vi "GF_CheckIgnoreError.vi"(1 "error in":errorcluster, 2 "Error code to ignore":i32) -> (0 "error out":errorcluster)   [LabVIEW 2016]
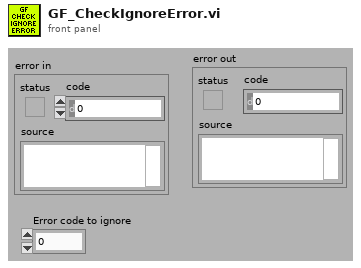
[diagram p1: front panel]
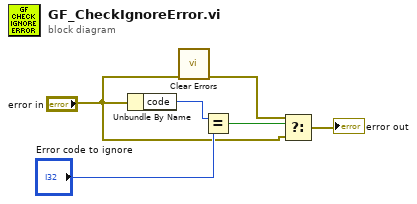
[diagram p0: block diagram]
diagram:
  n1 = Unbundle By Name("error in") -> ("code"=w6:i32)
  n2 = call <vilib>:"Clear Errors.vi"("error in (no error)"="error in") -> ("error out"=w3:errorcluster)  [unwired: 5 in, 1 out]
  n3 = Equal?(x=w6, y="Error code to ignore") -> (x = y?=w4:bool)
  n4 = Select(t=w3, s=w4, f="error in") -> (s? t:f=→"error out":errorcluster)
